vi "Controller.vi"(0 "Inputs":T3, 1 "Registers":T1={"Parameters"="Parameters", "VDCLinkToP_PISettings"="Range", "ID_to_VD_PISettings"="gains", "IQ_to_VQ_PISettings"="Setpoints", "VDCLink"="VDCLink", "P"="VDCLink", "Q"="VDCLink", "pf"="VDCLink"}, 11 "globalReset":bool) -> (4 "Outputs":T2)   [LabVIEW 2017, in "ActiveFrontEnd.lvlib"]
uses:
  ActiveFrontEnd.lvlib
  Inputs.ctl
  Outputs.ctl
  ControllerRegisters.ctl
  <vilib>/Utility/error.llb/Clear Errors.vi
  <vilib>/rvi/Emulation/niFpgaSctlEmulationGetInTimedLoop.vi
  <vilib>/rvi/DataTransferAndStorage/Container/Common/niFpgaContainerExecOnDevCompGetState.vi
  <vilib>/rvi/Emulation/niFpgaEmulationIsFPGAContextNoSignature.vi
  <vilib>/rvi/DataTransferAndStorage/Container/Common/niFpgaContainerGetUniqueNameForEmu.vi
  <vilib>/rvi/Memory/Memory_Emulation/niFpgaMemoryEmulationCacheClearOnFirstRun.vi
  <vilib>/rvi/Memory/Memory_Emulation/nirvimemoryEmulationManagerCache_MakeExclusive.vi
  <vilib>/rvi/Memory/Memory_Emulation/niFpgaMemoryEmulationValidateCache.vi
  <vilib>/rvi/Memory/Memory_Emulation/nirvimemoryEmulationManagerCache_InsertValue.vi
  <vilib>/rvi/Memory/Memory_Emulation/nirvimemoryEmulationManagerCache_ReleaseExclusive.vi
  <vilib>/rvi/Memory/Memory_Emulation/nirvimemoryEmulationManagerCache_GetValue.vi
  <vilib>/rvi/Memory/Memory_Emulation/nirvimemoryEmulationManagerCache_SetValue.vi
  <vilib>/rvi/Emulation/niFpgaProcessEmulError.vi
  <vilib>/rvi/DataTransferAndStorage/Container/XNode/niFpgaContainer.xnode
  <vilib>/rvi/DataTransferAndStorage/Register/Emulation/niFpgaRegisterEmulationRefIn.vi
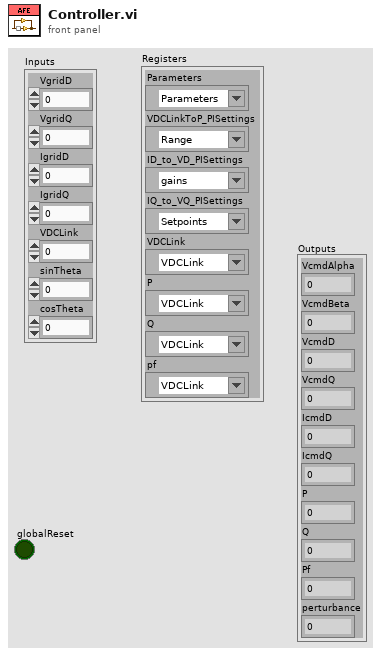
[diagram p1: front panel]
types:
  T1 = typedef "ActiveFrontEnd.lvlib/ControllerRegisters.ctl" = cluster{"Parameters":refnum<k21>, "VDCLinkToP_PISettings":refnum<k21>, "ID_to_VD_PISettings":refnum<k21>, "IQ_to_VQ_PISettings":refnum<k21>, "VDCLink":refnum<k21>, "P":refnum<k21>, "Q":refnum<k21>, "pf":refnum<k21>}
  T2 = typedef "ActiveFrontEnd.lvlib/Outputs.ctl" = cluster{"VcmdAlpha":sgl, "VcmdBeta":sgl, "VcmdD":sgl, "VcmdQ":sgl, "IcmdD":sgl, "IcmdQ":sgl, "P":sgl, "Q":sgl, "Pf":sgl, "perturbance":sgl}
  T3 = typedef "ActiveFrontEnd.lvlib/Inputs.ctl" = cluster{"VgridD":sgl, "VgridQ":sgl, "IgridD":sgl, "IgridQ":sgl, "VDCLink":sgl, "sinTheta":sgl, "cosTheta":sgl}
  T4 = cluster{"VDCLink_setpt":sgl, "VDCLinkRampRate":sgl, "Q_setpt":sgl, "Pf_setpt":sgl, "Mode":enum16{"Q Control", "Pf Control"}, "perturbance_amp":sgl, "perturbance_freq":sgl, "dT":sgl}
  T5 = cluster{"gains":cluster{"proportional gain":sgl, "integral gain":sgl}, "output range":cluster{"output high (Inf)":sgl, "output low (-Inf)":sgl}, "PI_state":enum8{"idle", "normal", "manual", "perturbance"}, "reset":bool, "manual":sgl}
  T6 = cluster{"gains":cluster{"proportional gain":sgl, "integral gain":sgl}, "output range":cluster{"output high (Inf)":sgl, "output low (-Inf)":sgl}, "PI_state":enum8{"idle", "normal", "manual", "perturbance"}, "reset":bool, "manual":sgl}[]
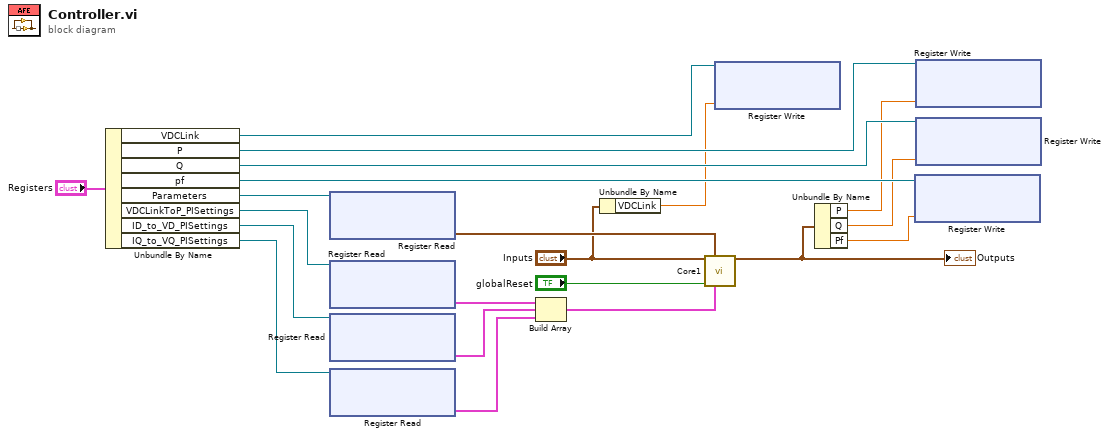
[diagram p0: block diagram]
diagram:
  n1 = Unbundle By Name("Registers") -> ("VDCLink"=w3:refnum<k21>, "P"=w10:refnum<k21>, "Q"=w9:refnum<k21>, "pf"=w8:refnum<k21>, "Parameters"=w20:refnum<k21>, "VDCLinkToP_PISettings"=w18:refnum<k21>, "ID_to_VD_PISettings"=w17:refnum<k21>, "IQ_to_VQ_PISettings"=w16:refnum<k21>)
  n2 = xnode ("Register Read")("Register In"=w20) -> ("Data"=w19:T4)  [unwired: 1 out]
  n3 = xnode ("Register Read")("Register In"=w18) -> ("Data"=w15:T5)  [unwired: 1 out]
  n4 = xnode ("Register Read")("Register In"=w17) -> ("Data"=w14:T5)  [unwired: 1 out]
  n5 = xnode ("Register Read")("Register In"=w16) -> ("Data"=w13:T5)  [unwired: 1 out]
  n6 = Build Array(w15, w14, w13) -> (w12:T6)
  n7 = Unbundle By Name("Inputs") -> ("VDCLink"=w2:sgl)
  n8 = call "Core1.vi"("Inputs"="Inputs", "Parameters"=w19, "globalReset"="globalReset", "PI_Settings"=w12) -> ("Outputs"=w11:T2)  [unwired: 11 in]
  "Outputs" <- w11
  n9 = xnode ("Register Write")("Data"=w2, "Register In"=w3) -> ()  [unwired: 1 out]
  n10 = Unbundle By Name(w11) -> ("P"=w7:sgl, "Q"=w6:sgl, "Pf"=w5:sgl)
  n11 = xnode ("Register Write")("Data"=w5, "Register In"=w8) -> ()  [unwired: 1 out]
  n12 = xnode ("Register Write")("Data"=w7, "Register In"=w10) -> ()  [unwired: 1 out]
  n13 = xnode ("Register Write")("Data"=w6, "Register In"=w9) -> ()  [unwired: 1 out]
